vi "Merge.vi"(8 "error in (no error)":errorcluster, 10 "YAML Parser in 2":refnum<class "YAML Parser.lvclass">, 11 "YAML Parser in":refnum<class "YAML Parser.lvclass">) -> (0 "error out":errorcluster, 3 "YAML Parser out":refnum<class "YAML Parser.lvclass">)   [LabVIEW 2015, in "YAML Parser.lvclass"]
uses:
  YAML Parser.lvclass
  YAML Parser.lvclass/YAML Parser.ctl
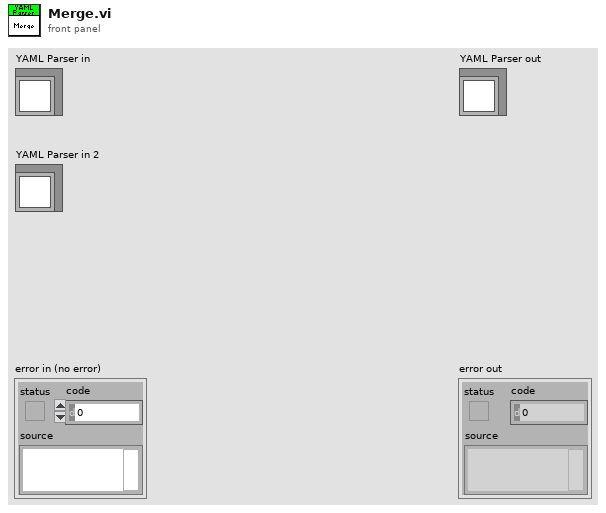
[diagram p1: front panel]
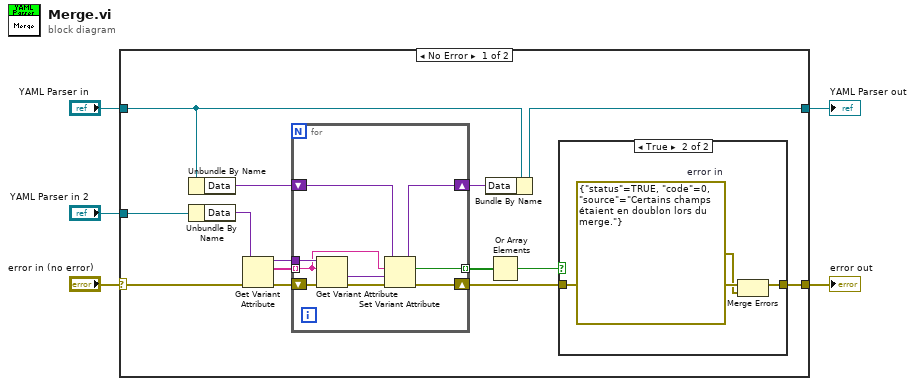
[diagram p0: block diagram]
diagram:
  n1 = case shown="No Error" "error in (no error)" {
    selector: "error in (no error)" -> [w16 w34]
    tunnel: [w6 w34] -> w4
    tunnel: [w10 w33] -> w2
    tunnel: "YAML Parser in" -> [w19 w33]
    tunnel: "YAML Parser in 2" -> [w18 _]
    frame No Error {
      n2 = Unbundle By Name(w19) -> ("Data"=w14:variant)
      n3 = Unbundle By Name(w18) -> ("Data"=w17:variant)
      n4 = Get Variant Attribute(Variant=w17, error in=w16) -> (duplicate Variant=w13:variant, names=w12:string[], error out=w15:errorcluster)  [unwired: 2 in, 1 out]
      n5 = for {
        shift-right: [w31] -> w9
        shift-left: w14 -> [w32]
        shift-right: [w28] -> w7
        shift-left: w15 -> [w30]
        tunnel: w13 -> [w27]
        tunnel: w12 -> [w26] mode=indexing
        tunnel: [w24] -> w11 mode=indexing
        n6 = Get Variant Attribute(Variant=w27, name=w26, error in=w30) -> (value=w25:variant, error out=w29:errorcluster)  [unwired: 1 in, 2 out]
        n7 = Set Variant Attribute(Variant=w32, name=w26, value=w25, error in=w29) -> (Variant out=w31:variant, replaced=w24:bool, error out=w28:errorcluster)
      }
      n8 = Bundle By Name(cluster=w19, "Data"=w9) -> (w10:refnum<class "YAML Parser.lvclass">)
      n9 = Or Array Elements(Boolean array=w11) -> (logical OR=w8:bool)
      n10 = case shown="True" w8 {
        tunnel: w7 -> [w20 w23]
        tunnel: [w20 w22] -> w6
        frame False {
        }
        frame True {
          w21 = errorcluster {"status"=TRUE, "code"=0, "source"="Certains champs étaient en doublon lors du merge."}  # error in
          n11 = Merge Errors(w23, w21) -> (w22:errorcluster)
        }
      }
    }
    frame Error {
    }
  }
  "error out" <- w4
  "YAML Parser out" <- w2
